vi "BufferAndTrigger.vi"(0 "Logging Configuration":T2={"Log File Base Path"=path "", "Samples to Save"=0, "Trigger - Threshold"=0.0, "Trigger - Channel"=0, "Always Log"=FALSE, "External Trigger"=FALSE, "External Trigger Armed"=FALSE, "TDMS File Reference"=refnum, "DAQVersion"="", "SWVersion"="", "CircSamples"=0, "BeepWhenComplete"=FALSE, "ChannelConfig"=[], "ActiveChannels"=[], "Title"="", "Description"="", "ChannelNames"=[], "ResponseExtension"=TRUE}, 1 "State":T1={"State"=enum."Not Logging", "Samples to Save"=0, "Force Trigger"=FALSE}, 2 "WaveformIN":waveform(dbl)[](array[waveform]), 3 "error in (no error)":errorcluster) -> (5 "TriggerTimeStamp":timestamp=timestamp(3569548862.6211414 s since 1904-01-01), 6 "Logging Configuration Out":T2={"Log File Base Path"=path "", "Samples to Save"=0, "Trigger - Threshold"=0.0, "Trigger - Channel"=0, "Always Log"=FALSE, "External Trigger"=FALSE, "External Trigger Armed"=FALSE, "TDMS File Reference"=refnum, "DAQVersion"="", "SWVersion"="", "CircSamples"=0, "BeepWhenComplete"=FALSE, "ChannelConfig"=[], "ActiveChannels"=[], "Title"="", "Description"="", "ChannelNames"=[], "ResponseExtension"=TRUE}, 7 "WaveformOUT":waveform(dbl)[](array[waveform]), 8 "TriggerIndex":i32, 9 "Trigger":bool, 10 "error out":errorcluster)   [LabVIEW 2017, in "Logging.lvlib"]
doc: "Given the Logging Configuration, Waveform Data, and Force Trigger information, return true if a trigger has been detected."
uses:
  Logging.lvlib
  Logging Configuration.ctl
  Logging State.ctl
  <userlib>/Circular Buffer/Controls/Circular Buffer Operations.ctl
  <vilib>/Waveform/WDTOps.llb/WDT Number of Waveform Samples DBL.vi
  <userlib>/Circular Buffer/Instance VIs/Circular Buffer(2D Wfm with Attributes).vi
  <userlib>/Circular Buffer/Circular Buffer.lvlib
  <vilib>/Analysis/NI_AALPro.lvlib
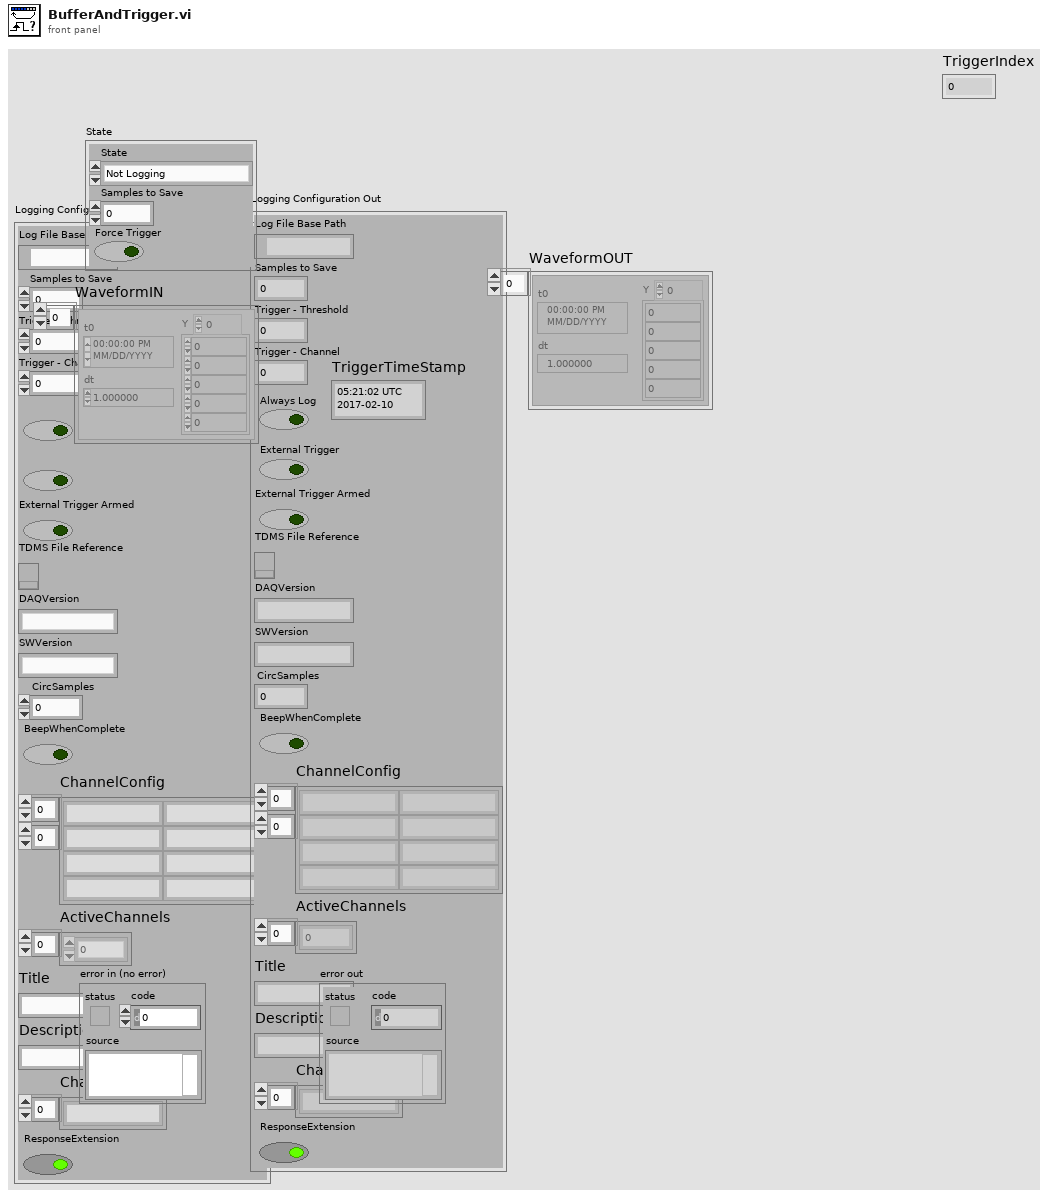
[diagram p1: front panel]
types:
  T1 = typedef "Logging.lvlib/Logging State.ctl" = cluster{"State":enum16{"Logging", "Not Logging"}, "Samples to Save":u32, "Force Trigger":bool}
  T2 = typedef "Logging.lvlib/Logging Configuration.ctl" = cluster{"Log File Base Path":path, "Samples to Save":u32, "Trigger - Threshold":dbl, "Trigger - Channel":u32, "Always Log":bool, "External Trigger":bool, "External Trigger Armed":bool, "TDMS File Reference":refnum<k34>, "DAQVersion":string, "SWVersion":string, "CircSamples":u32, "BeepWhenComplete":bool, "ChannelConfig":string[][], "ActiveChannels":i32[], "Title":string, "Description":string, "ChannelNames":string[], "ResponseExtension":bool}
  T3 = typedef "Circular Buffer.lvlib/Circular Buffer Operations.ctl" = enum16{"Initialize", "Get Backlog", "Write", "Read (continuous)", "Read (most recent)", "Peak"}
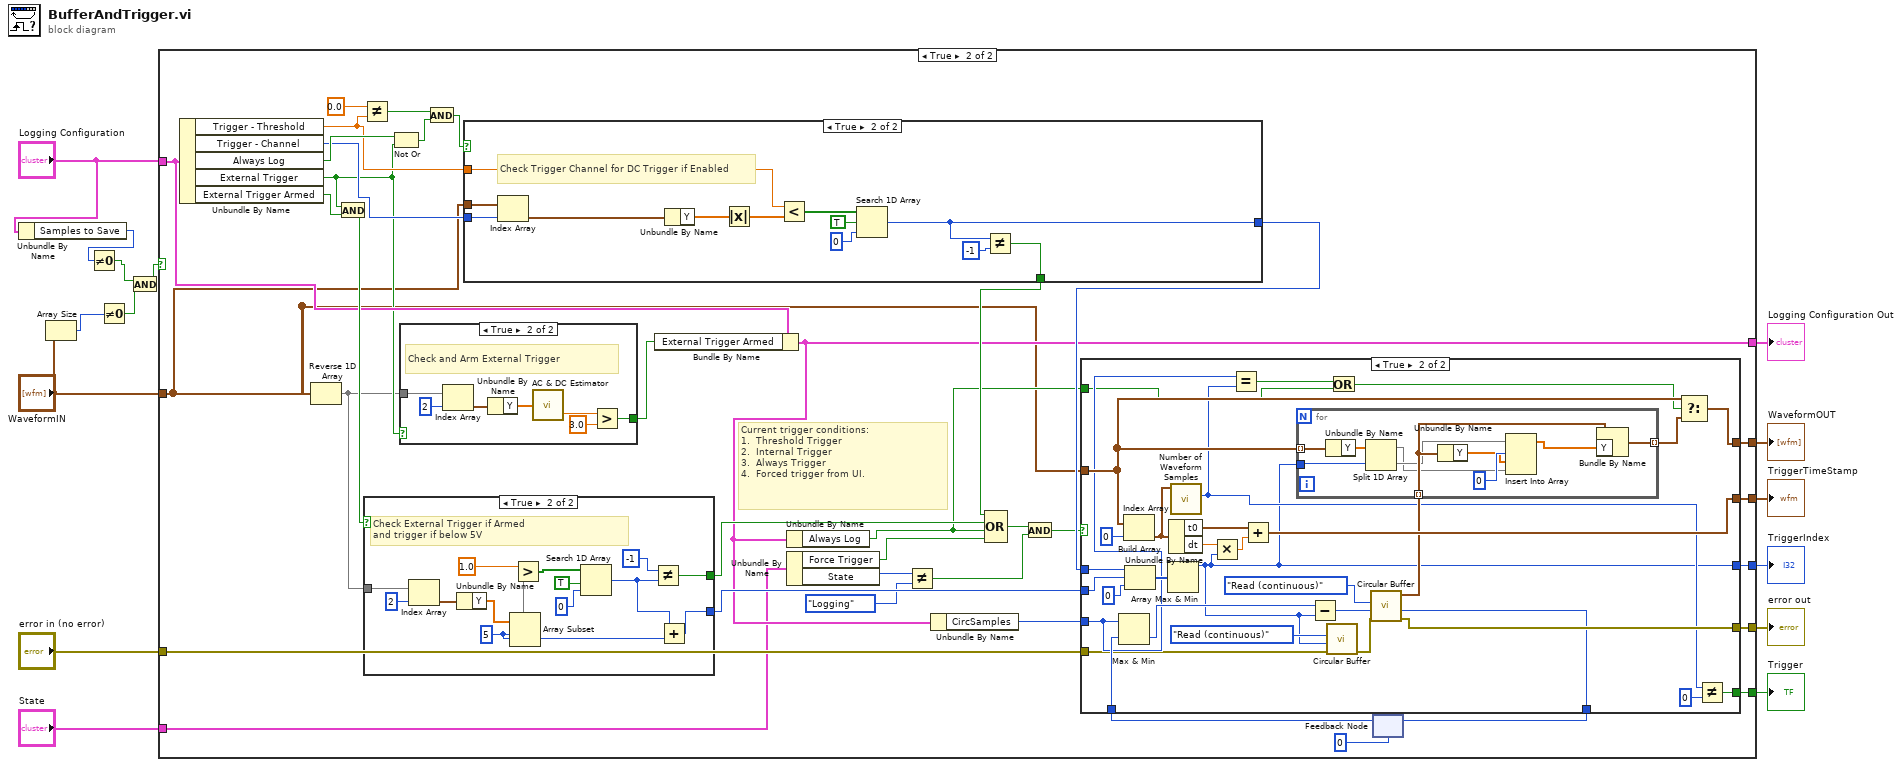
[diagram p0: block diagram]
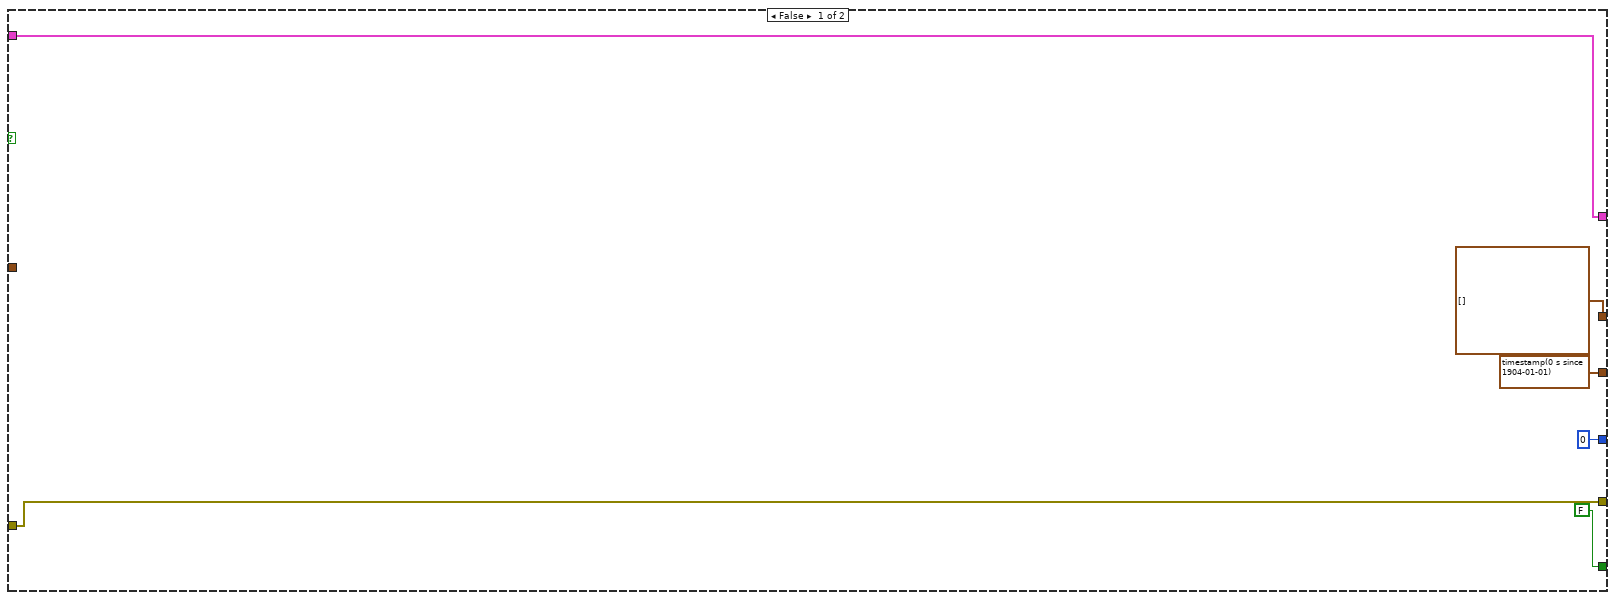
[diagram p2: hidden frame]
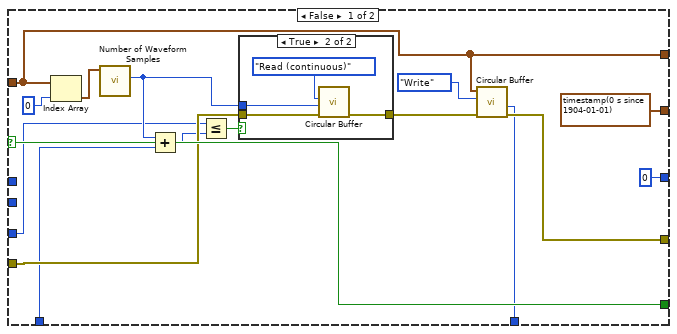
[diagram p3: hidden frame]
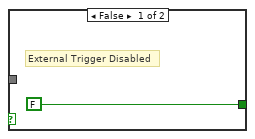
[diagram p5: hidden frame]
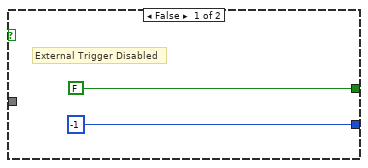
[diagram p6: hidden frame]
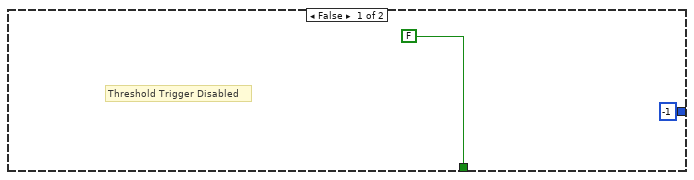
[diagram p7: hidden frame]
diagram:
  n1 = Unbundle By Name("Logging Configuration") -> ("Samples to Save"=w7:u32)
  n2 = Array Size(array="WaveformIN") -> (size(s)=w3:i32)
  n3 = Not Equal To 0?(x=w7) -> (x != 0?=w5:bool)
  n4 = Not Equal To 0?(x=w3) -> (x != 0?=w4:bool)
  n5 = And(x=w5, y=w4) -> (x .and. y?=w1:bool)
  n6 = case shown="True" w1 {
    tunnel: [timestamp(0 s since 1904-01-01) w46] -> w15
    tunnel: [waveform(dbl)[] [] ("WaveformIN") w45] -> w14
    tunnel: "WaveformIN" -> [_ w23]
    tunnel: [FALSE w42] -> w13
    tunnel: [w21 w41] -> w12
    tunnel: "error in (no error)" -> [w21 w37]
    tunnel: [w17 w40] -> w10
    tunnel: "Logging Configuration" -> [w17 w39]
    tunnel: "State" -> [_ w33]
    tunnel: [0 w24] -> w6
    frame False {
    }
    frame True {
      # "Current trigger conditions:\n1.  Threshold Trigger\n2.  Internal Trigger\n3.  Always Trigger\n4.  Forced trigger from UI."
      n7 = Unbundle By Name(w39) -> ("Trigger - Threshold"=w48:dbl, "Trigger - Channel"=w49:u32, "Always Log"=w50:bool, "External Trigger"=w26:bool, "External Trigger Armed"=w25:bool)
      n8 = Reverse 1D Array(array=w23) -> (reversed array=w22:waveform(dbl)[])
      n9 = And(x=w26, y=w25) -> (x .and. y?=w51:bool)
      n10 = Not Equal?(x=0.0 ("y"), y=w48) -> (x != y?=w54:bool)
      n11 = case shown="True" w51 {
        tunnel: w22 -> [_ w144]
        tunnel: [FALSE w141] -> w56
        tunnel: [-1 w133] -> w43
        frame False {
          # "External Trigger Disabled"
        }
        frame True {
          w132 = 5 ("index")
          # "Check External Trigger if Armed\nand trigger if below 5V"
          n12 = Index Array(array=w144, index=2) -> (element=w143:waveform(dbl))
          n13 = Unbundle By Name(w143) -> ("Y"=w135:dbl[])
          n14 = Array Subset(array=w135, index=w132) -> (w131:dbl[])  [unwired: 1 in]
          n15 = Greater?(x=1.0 ("y"), y=w131) -> (0:w140:bool[])
          n16 = Search 1D Array(1D array=w140, element=TRUE, start index (0)=0) -> (index of element=w134:i32)
          n17 = Not Equal?(x=-1, y=w134) -> (x != y?=w141:bool)
          n18 = Add(x=w134, y=w132) -> (x+y=w133:i32)
        }
      }
      n19 = Not Or(1:w26, 2:w50) -> (0:w57:bool)
      n20 = case shown="True" w26 {
        tunnel: w22 -> [_ w125]
        tunnel: [FALSE w126] -> w52
        frame False {
          # "External Trigger Disabled"
        }
        frame True {
          # "Check and Arm External Trigger"
          n21 = Index Array(array=w125, index=2) -> (element=w124:waveform(dbl))
          n22 = Unbundle By Name(w124) -> ("Y"=w128:dbl[])
          n23 = call <vilib>:"AC & DC Estimator.vi"("Signal (V)"=w128) -> ("DC estimate (V)"=w127:dbl)  [unwired: 1 out]
          n24 = Greater?(x=w127, y=3.0) -> (0:w126:bool)
        }
      }
      n25 = And(x=w54, y=w57) -> (x .and. y?=w55:bool)
      n26 = case shown="True" w55 {
        tunnel: w23 -> [_ w150]
        tunnel: [FALSE w151] -> w58
        tunnel: w48 -> [_ w157]
        tunnel: w49 -> [_ w149]
        tunnel: [-1 w153] -> w44
        frame False {
          # "Threshold Trigger Disabled"
        }
        frame True {
          # "Check Trigger Channel for DC Trigger if Enabled"
          n27 = Index Array(array=w150, index=w149) -> (element=w158:waveform(dbl))
          n28 = Unbundle By Name(w158) -> ("Y"=w148:dbl[])
          n29 = Absolute Value(x=w148) -> (abs(x)=w147:dbl[])
          n30 = Less?(x=w157, y=w147) -> (x < y?=w156:bool[])
          n31 = Search 1D Array(1D array=w156, element=TRUE, start index (0)=0) -> (index of element=w153:i32)
          n32 = Not Equal?(x=w153, y=-1) -> (x != y?=w151:bool)
        }
      }
      n33 = Bundle By Name(cluster=w39, "External Trigger Armed"=w52) -> (w40:T2)
      n34 = Unbundle By Name(w40) -> ("Always Log"=w27:bool)
      n35 = Unbundle By Name(w33) -> ("Force Trigger"=w53:bool, "State"=w31:enum16{"Logging", "Not Logging"})
      n36 = Not Equal?(x=w31, y=enum16{"Logging", "Not Logging"}."Logging" ("x")) -> (x != y?=w30:bool)
      n37 = Unbundle By Name(w40) -> ("CircSamples"=w38:u32)
      n38 = Compound Arithmetic op=OR(w58, w56, w27, w53) -> (w29:bool)
      n39 = And(x=w29, y=w30) -> (x .and. y?=w28:bool)
      n40 = feedback #1(0 ("Elements Remaining")) -> (w34:i32)
      n41 = case shown="True" w28 {
        selector: w28 -> [w73 _]
        tunnel: w23 -> [w67 w92]
        tunnel: [timestamp(0 s since 1904-01-01) w105] -> w46
        tunnel: [w67 w90] -> w45
        tunnel: w44 -> [_ w104]
        tunnel: w43 -> [_ w103]
        tunnel: [w73 w101] -> w42
        tunnel: [w68 w97] -> w41
        tunnel: w37 -> [w66 w82]
        tunnel: w34 -> [w63 w93]
        tunnel: [w65 w95] -> w35
        tunnel: w38 -> [w62 w88]
        tunnel: w27 -> [_ w86]
        tunnel: [0 w80] -> w24
        frame False {
          n42 = Index Array(array=w67, index=0) -> (element=w72:waveform(dbl))
          n43 = call-poly <vilib>:"Number of Waveform Samples.vi"("waveform in"=w72) -> ("number of samples"=w64:i32)  [unwired: 8 in, 2 out]
          n44 = Add(x=w64, y=w63) -> (x+y=w61:i32)
          n45 = Less Or Equal?(x=w62, y=w61) -> (x <= y?=w60:bool)
          n46 = case shown="True" w60 {
            tunnel: w64 -> [_ w78]
            tunnel: w66 -> [w75 w77]
            tunnel: [w75 w76] -> w71
            frame False {
            }
            frame True {
              n47 = call-poly <userlib>:"Circular Buffer.vi"("error in (no error)"=w77, "Read Size"=w78, "Operation"=Circular_Buffer_Operations."Read (continuous)") -> ("error out"=w76:errorcluster)  [unwired: 5 in, 3 out]
            }
          }
          n48 = call-poly <userlib>:"Circular Buffer.vi"("error in (no error)"=w71, "Operation"=Circular_Buffer_Operations."Write", "Data In"=w67) -> ("error out"=w68:errorcluster, "Elements Remaining"=w65:i32)  [unwired: 5 in, 2 out]
        }
        frame True {
          n49 = Max & Min(x=w88, y=w93) -> (min(x,y)=w94:u32)  [unwired: 1 out]
          n50 = Index Array(array=w92, index=0) -> (element=w99:waveform(dbl))
          n51 = Build Array(w104, w103, 0 ("element")) -> (w109:i32[])
          n52 = Array Max & Min(array=w109) -> (max value=w80:i32)  [unwired: 3 out]
          n53 = Unbundle By Name(w99) -> ("t0"=w108:timestamp, "dt"=w107:dbl)
          n54 = call-poly <vilib>:"Number of Waveform Samples.vi"("waveform in"=w99) -> ("number of samples"=w89:i32)  [unwired: 8 in, 2 out]
          n55 = Multiply(x=w107, y=w80) -> (x*y=w106:dbl)
          n56 = Equal?(x=w88, y=w89) -> (x = y?=w87:bool)
          n57 = Add(x=w108, y=w106) -> (x+y=w105:timestamp)
          n58 = Subtract(x=w94, y=w80) -> (x-y=w84:u32)
          n59 = call-poly <userlib>:"Circular Buffer.vi"("error in (no error)"=w82, "Read Size"=w80, "Operation"=Circular_Buffer_Operations."Read (continuous)") -> ("error out"=w81:errorcluster)  [unwired: 5 in, 3 out]
          n60 = Or(x=w87, y=w86) -> (x .or. y?=w85:bool)
          n61 = call-poly <userlib>:"Circular Buffer.vi"("error in (no error)"=w81, "Read Size"=w84, "Operation"=Circular_Buffer_Operations."Read (continuous)") -> ("error out"=w97:errorcluster, "Elements Remaining"=w95:i32, "Data Out"=w96:waveform(dbl)[])  [unwired: 5 in, 1 out]
          n62 = for {
            tunnel: w92 -> [w117] mode=indexing
            tunnel: [w120] -> w91 mode=indexing
            tunnel: w80 -> [w118]
            tunnel: w96 -> [w116] mode=indexing
            n63 = Unbundle By Name(w117) -> ("Y"=w119:dbl[])
            n64 = Split 1D Array(array=w119, index=w118) -> (first subarray=w112:dbl[], second subarray=w115:dbl[])
            n65 = Unbundle By Name(w116) -> ("Y"=w113:dbl[])
            n66 = Insert Into Array(array=w115, index=0, new element #1=w113, new element #2=w112) -> (w111:dbl[])
            n67 = Bundle By Name(cluster=w116, "Y"=w111) -> (w120:waveform(dbl))
          }
          n68 = Select(t=w92, s=w85, f=w91) -> (s? t:f=w90:waveform(dbl)[])
          n69 = Not Equal?(x=w89, y=0) -> (x != y?=w101:bool)
        }
      }
      n70 = feedback-in #1(w35) -> ()
    }
  }
  "Trigger" <- w13
  "Logging Configuration Out" <- w10
  "error out" <- w12
  "TriggerTimeStamp" <- w15
  "WaveformOUT" <- w14
  "TriggerIndex" <- w6
